vi "Tools_KeyedArray Index Wildcards.vi"(4 "case matching (sensitive)":T1=enum."system", 5 "default value":string, 6 "key":string, 7 "array in":T2) -> (0 "match pattern":string, 1 "found pattern":bool, 2 "value":string, 3 "duplicate array":T2)   [LabVIEW 2012]
doc: "Returns the value of the first element whose key, treated like wildcard expressions, matches <B>key</B>."
uses:
  Tools_KeyedArray KeyedArray.ctl
  String/Tools_String Case Matching.ctl
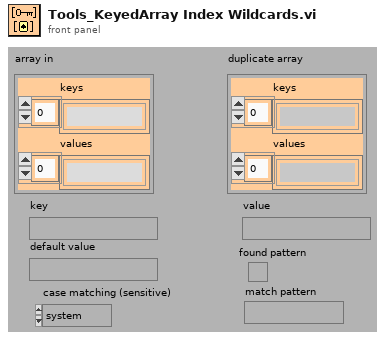
[diagram p1: front panel]
types:
  T1 = typedef "Tools_String Case Matching.ctl" = enum16{"a != A", "a == A", "system"}
  T2 = typedef "Tools_KeyedArray KeyedArray.ctl" = cluster{"keys":string[], "values":string[]}
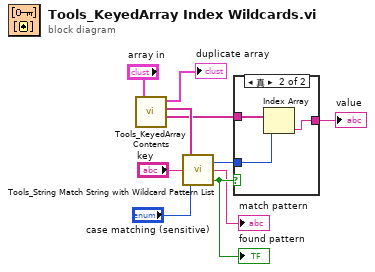
[diagram p0: block diagram]
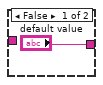
[diagram p2: hidden frame]
diagram:
  n1 = call "Tools_KeyedArray Contents.vi"("array in"="array in") -> ("values"=w6:string[], "keys"=w9:string[], "duplicate array"=→"duplicate array":T2)  [unwired: 4 out]
  n2 = call "Tools_String Match String with Wildcard Pattern List.vi"("case matching (sensitive)"="case matching (sensitive)", "string"="key", "pattern list"=w9) -> ("found substring"=w7:bool, "match pattern"=→"match pattern":string, "index"=w5:i32)
  "found pattern" <- w7
  n3 = case shown="真" w7 {
    tunnel: w6 -> [_ w14]
    tunnel: w5 -> [_ w13]
    tunnel: ["default value" w12] -> w4
    frame False {
    }
    frame True {
      n4 = Index Array(array=w14, index=w13) -> (element=w12:string)
    }
  }
  "value" <- w4
